vi "State_Manager.vi"(0 "Mode":enum16{"Initialize", "Manage", "Close"}(ring), 1 "Clear queue":bool, 3 "Immediate actions":bool[](array[boolean]), 4 "Reset":bool[](array[boolean]), 5 "Auto actions":bool[](array[boolean]), 6 "Config file name":path=path "C:/Users/ceslab/Documents/CES LabView/Configuration/CES_Config_test.ini", 7 "Abort action":bool) -> (8 "Spectrum type":u32, 9 "Substate":string, 10 "Action Queue":string[](array[string]), 12 "Action list":string[](array[string]), 13 "Action times":cluster{dbl[], dbl[]} {"?" format="%.2f"; "?" format="%.2f"}, 14 "Output cluster":T1, 17 "Current state":i32, 18 "Time left":dbl, 19 "error out":errorcluster)   [LabVIEW 2025]
uses:
  <vilib>/regexp/Match Regular Expression.xnode
panel:
  out "State array":i32[][](array[numeric])
  out "Action data":i32[][](array[numeric])
  out "Action count":i32[](array[numeric])
  out "Linked index":i32[](array[numeric])
  out "Mode":i32[](array[numeric])
  out "Frequency":i32[](array[numeric])
  out "Linked state":string[](array[string])
  out "Action Queue":i32[](array[numeric])
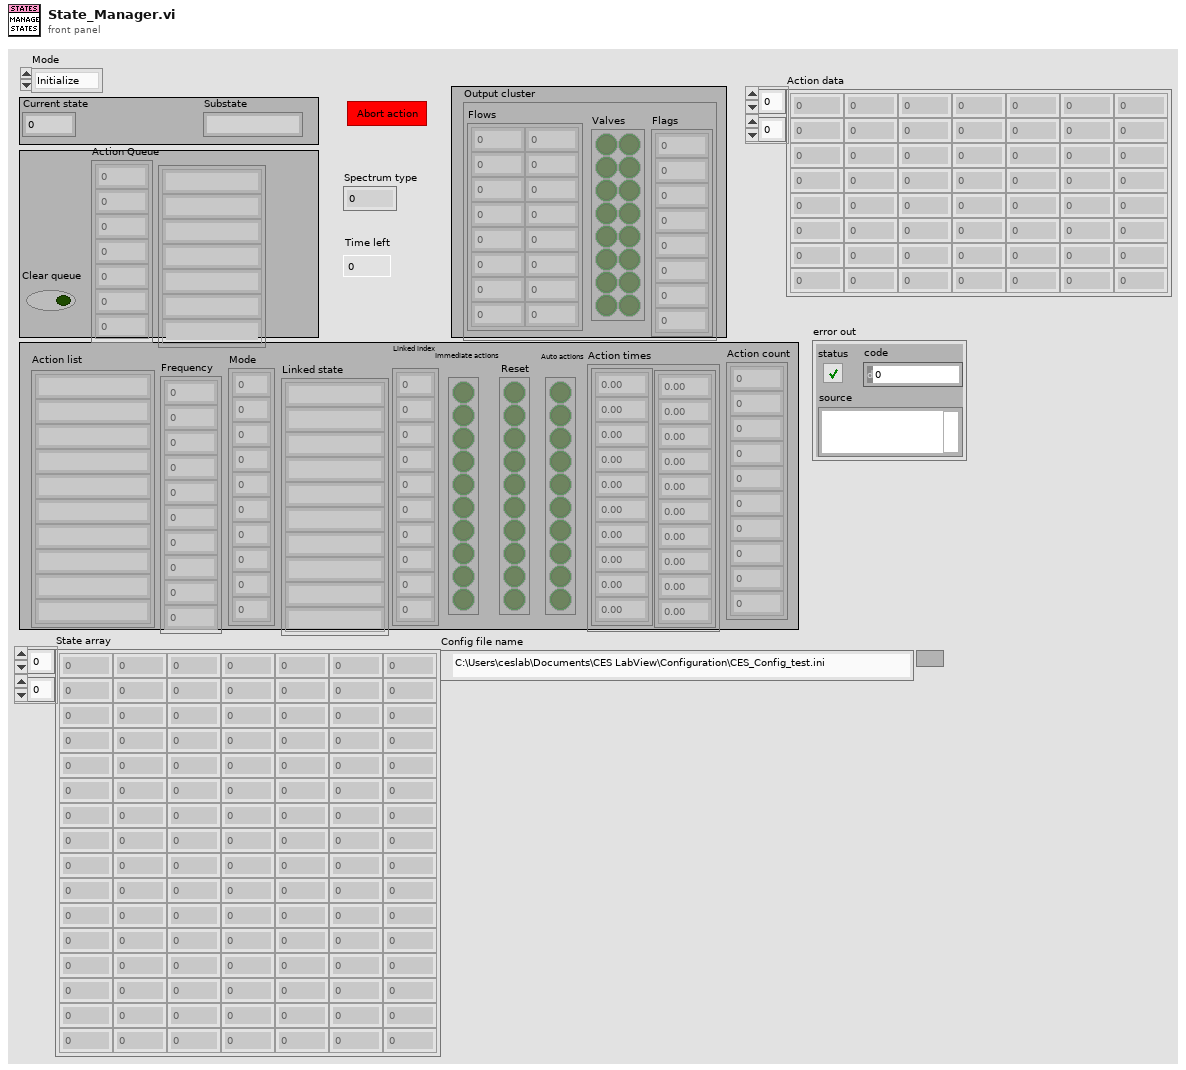
[diagram p1: front panel]
types:
  T1 = cluster{"Flows":dbl[][], "Valves":bool[][], "Flags":i32[]}
  T2 = enum16{"Spectrometer", "Calculations", "BBB", "States", "Actions"}
  T3 = cluster{"num_flags":i32, "num_flows":i32, "num_valves":i32}
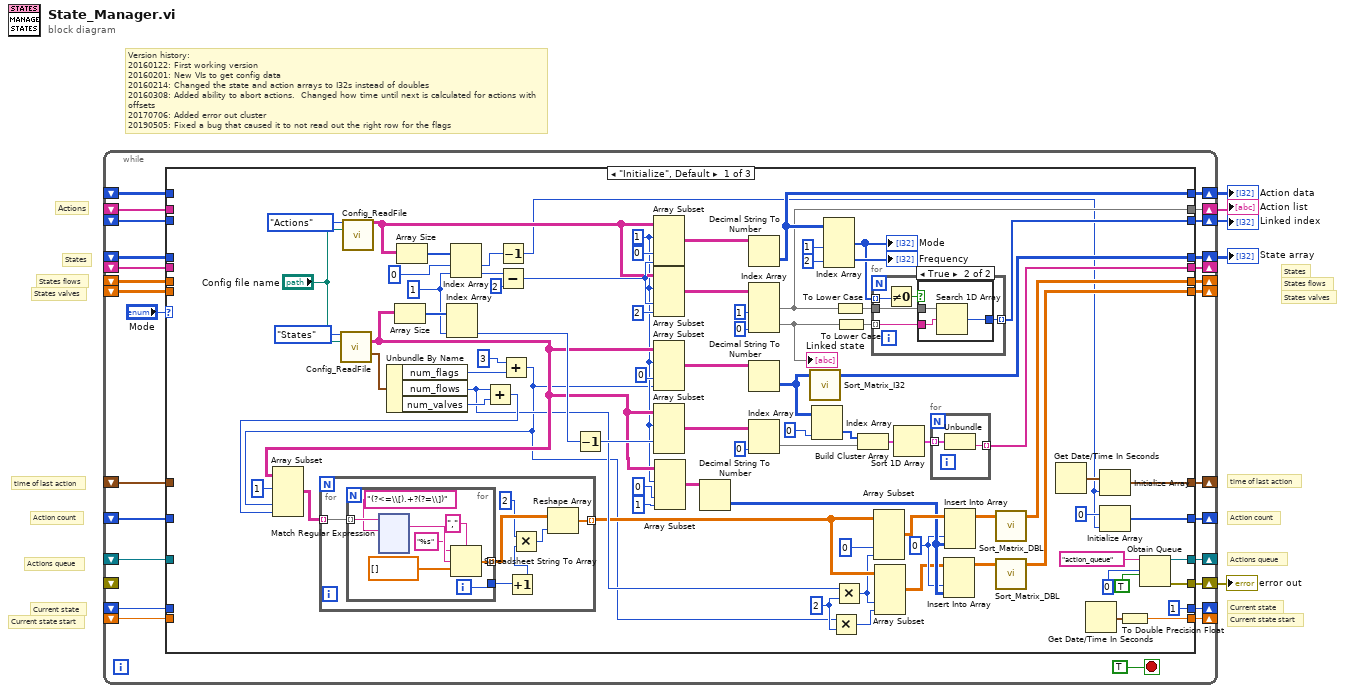
[diagram p0: block diagram]
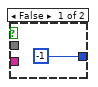
[diagram p2: hidden frame]
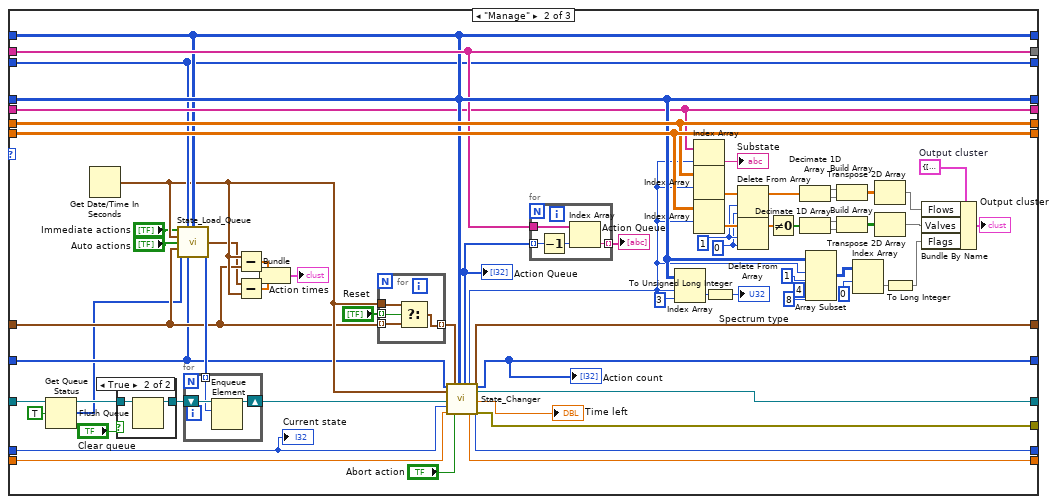
[diagram p3: hidden frame]
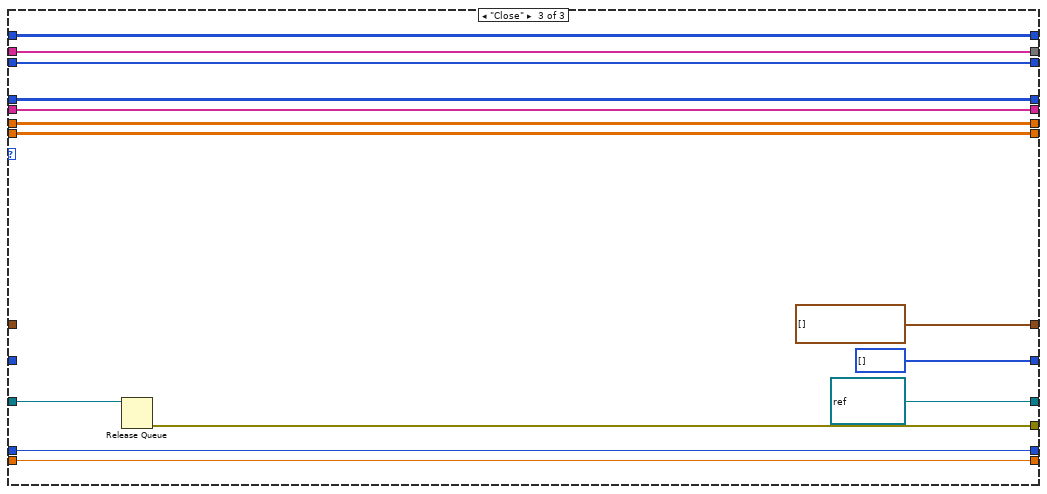
[diagram p5: hidden frame]
diagram:
  # "Version history:\n20160122: First working version\n20160201: New VIs to get config data\n20160214: Changed the state and action arrays to I32s instead of doubles\n20160308: Added ability to abort actions.  Changed how time until next is calculated for actions with offsets\n20170706: Added error out cluster\n20190505: Fixed a bug that caused it to not read out the right row for the flags"
  # "Action count"
  # "Current state start"
  # "Current state"
  # "time of last action"
  # "Actions queue"
  # "States valves"
  # "States flows"
  # "States"
  # "Actions"
  # "Action count"
  # "Current state start"
  # "Current state"
  # "time of last action"
  # "Actions queue"
  # "States valves"
  # "States flows"
  # "States"
  n1 = while {
    shift-right: [w30] -> w3
    shift-left: _ -> [w29]
    shift-right: [w28] -> w5
    shift-left: _ -> [w27]
    shift-right: [w17] -> w2
    shift-left: _ -> [w21]
    shift-right: [w26] -> _
    shift-left: _ -> [w20]
    shift-right: [w25] -> _
    shift-left: _ -> [w19]
    shift-right: [w24] -> _
    shift-left: _ -> [w18]
    shift-right: [w23] -> _
    shift-left: _ -> [w22]
    shift-right: [w16] -> _
    shift-left: _ -> [w15]
    shift-right: [w14] -> _
    shift-left: _ -> [w13]
    shift-right: [w12] -> w4
    shift-left: _ -> [w11]
    shift-right: [w9] -> _
    shift-left: _ -> [w7]
    shift-right: [w10] -> _
    shift-left: _ -> [w8]
    shift-right: [w6] -> w1
    shift-left: _ -> [_]
    stop <- TRUE stop-if-true
    n2 = case shown="\"Initialize\", Default" "Mode" {
      tunnel: [w91 w275 w352] -> w30
      tunnel: w29 -> [_ w275 w352]
      tunnel: [w81 w285 w351] -> w28
      tunnel: w27 -> [_ w285 w351]
      tunnel: [w100 w277 w349] -> w26
      tunnel: [w75 w317 w348] -> w25
      tunnel: [w74 w318 w347] -> w24
      tunnel: [w99 w282 timestamp[] []] -> w23
      tunnel: w22 -> [_ w269 _]
      tunnel: w21 -> [_ w286 w350]
      tunnel: w20 -> [_ w277 w349]
      tunnel: w19 -> [_ w317 w348]
      tunnel: w18 -> [_ w318 w347]
      tunnel: [w76 w286 w350] -> w17
      tunnel: [w95 w283 refnum<queue> refnum ("queue out")] -> w16
      tunnel: w15 -> [_ w323 w346]
      tunnel: [w92 w278 i32[] []] -> w14
      tunnel: w13 -> [_ w268 _]
      tunnel: [w85 w274 w342] -> w12
      tunnel: w11 -> [_ w274 w342]
      tunnel: [1 w260 w341] -> w10
      tunnel: [w82 w261 w340] -> w9
      tunnel: w8 -> [_ w280 w341]
      tunnel: w7 -> [_ w281 w340]
      tunnel: [w70 w259 w339] -> w6
      frame "Initialize", Default {
        w42 = 0 ("disabled index (col)")
        w39 = 2 ("y")
        w58 = 1 ("index")
        w50 = 1 ("index")
        n3 = call "Config_ReadFile.vi"("Section"=T2."States", "Config file name"="Config file name") -> ("State data"=w54:string[][], "state_elements"=w62:T3)  [unwired: 7 in, 5 out]
        n4 = call "Config_ReadFile.vi"("Section"=T2."Actions", "Config file name"="Config file name") -> ("Actions data"=w68:string[][])  [unwired: 7 in, 6 out]
        n5 = Unbundle By Name(w62) -> ("num_flags"=w61:i32, "num_flows"=w46:i32, "num_valves"=w49:i32)
        n6 = Array Size(array=w54) -> (size(s)=w69:i32[])
        n7 = Array Size(array=w68) -> (size(s)=w67:i32[])
        n8 = Index Array(array=w69, index #2=w58) -> (element #2=w57:i32)  [unwired: 1 in, 1 out]
        n9 = Index Array(array=w67, index #1=0 ("index"), index #2=w58) -> (element #1=w64:i32, element #2=w66:i32)
        n10 = Add(x=w46, y=w49) -> (x+y=w48:i32)
        n11 = Decrement(x=w64) -> (x-1=w63:i32)
        n12 = Subtract(x=w66, y=2 ("index")) -> (x-y=w72:i32)
        n13 = Add(x=3, y=w61) -> (x+y=w38:i32)
        n14 = Array Subset(array=w54, index (row)=1 ("index"), index (col)=w38, length (col)=w48) -> (w55:string[][])  [unwired: 1 in]
        n15 = for {
          tunnel: w55 -> [w121] mode=indexing
          tunnel: [w115] -> w41 mode=indexing
          n16 = for {
            tunnel: w121 -> [w129] mode=indexing
            tunnel: [w123] -> w120 mode=indexing
            tunnel: [w122] -> w116
            i -> [w122]
            n17 = xnode "Match Regular Expression"("input string"=w129, "regular expression"="(?<=\\[).+?(?=\\])") -> ("whole match"=w127:string)  [unwired: 4 in, 4 out]
            n18 = Spreadsheet String To Array(delimiter (Tab)=",", format string="%s" ("spreadsheet string"), spreadsheet string=w127, array type (2D Dbl)=dbl[] []) -> (array=w123:dbl[])
          }
          n19 = Increment(x=w116) -> (x+1=w117:i32)
          n20 = Multiply(x=2, y=w117) -> (x*y=w118:i32)
          n21 = Reshape Array(w120, w118) -> (w115:dbl[])
        }
        n22 = Decrement(x=w57) -> (x-1=w71:i32)
        n23 = Array Subset(array=w68, index (row)=w50, index (col)=0 ("index"), length (col)=w72) -> (w109:string[][])  [unwired: 1 in]
        n24 = Array Subset(array=w68, index (row)=w50, index (col)=w72, length (col)=2 ("length")) -> (w107:string[][])  [unwired: 1 in]
        n25 = Array Subset(array=w54, index (row)=w50, index (col)=0 ("index"), length (col)=w38) -> (w113:string[][])  [unwired: 1 in]
        n26 = Array Subset(array=w54, index (row)=w50, index (col)=w71) -> (w112:string[][])  [unwired: 2 in]
        n27 = Array Subset(array=w54, index (row)=w50, index (col)=0 ("index"), length (col)=1 ("length")) -> (w51:string[][])  [unwired: 1 in]
        n28 = Decimal String To Number(string=w51) -> (number=w43:i32[][])  [unwired: 2 in, 1 out]
        n29 = Decimal String To Number(string=w109) -> (number=w91:i32[][])  [unwired: 2 in, 1 out]
        n30 = Index Array(array=w107, index (col) #1=1 ("disabled index (col)"), index (col) #2=0 ("disabled index (col)")) -> (element #1=w81:string[], element #2=w79:string[])  [unwired: 2 in]
        "Linked state" <- w79
        n31 = Decimal String To Number(string=w113) -> (number=w77:i32[][])  [unwired: 2 in, 1 out]
        n32 = Index Array(array=w112, index (col)=0 ("disabled index (col)")) -> (element=w103:string[])  [unwired: 1 in]
        n33 = call "Sort_Matrix_I32.vi"("Unsort array in"=w77) -> ("Sorted array out"=w76:i32[][])  [unwired: 26 in]
        n34 = Index Array(array=w77, index (col)=0 ("disabled index (col)")) -> (element=w104:i32[])  [unwired: 1 in]
        n35 = Index Array(array=w91, index (col) #1=1 ("disabled index (col)"), index (col) #2=2 ("disabled index (col)")) -> (element #1=w86:i32[], element #2=→"Frequency":i32[])  [unwired: 2 in]
        "Mode" <- w86
        n36 = Multiply(x=w38, y=w39) -> (x*y=w37:i32)
        n37 = Multiply(x=w46, y=w39) -> (x*y=w40:i32)
        n38 = To Lower Case(string=w81) -> (all lower case string=w80:string[])
        n39 = To Lower Case(string=w79) -> (all lower case string=w78:string[])
        n40 = Build Cluster Array(w104, w103) -> (w102:cluster{"Section":i32, "Section":string}[])
        n41 = for {
          tunnel: w78 -> [w249] mode=indexing
          tunnel: w86 -> [w251] mode=indexing
          tunnel: w80 -> [w248]
          tunnel: [w247] -> w85 mode=indexing
          n42 = Not Equal To 0?(x=w251) -> (x != 0?=w250:bool)
          n43 = case shown="True" w250 {
            tunnel: w249 -> [_ w254]
            tunnel: w248 -> [_ w255]
            tunnel: [-1 w253] -> w247
            frame False {
            }
            frame True {
              n44 = Search 1D Array(1D array=w255, element=w254) -> (index of element=w253:i32)  [unwired: 1 in]
            }
          }
        }
        n45 = Array Subset(array=w41, index (col)=0 ("index"), length (col)=w40) -> (w45:dbl[][])  [unwired: 2 in]
        n46 = Array Subset(array=w41, index (col)=w40, length (col)=w37) -> (w36:dbl[][])  [unwired: 2 in]
        n47 = Sort 1D Array(array=w102) -> (sorted array=w101:cluster{"Section":i32, "Section":string}[])
        n48 = for {
          tunnel: w101 -> [w257] mode=indexing
          tunnel: [w256] -> w100 mode=indexing
          n49 = Unbundle(w257) -> ("Section"=w256:string)  [unwired: 1 out]
        }
        n50 = Insert Into Array(array=w36, index (col)=w42, new element=w43) -> (w35:dbl[][])  [unwired: 1 in]
        n51 = Insert Into Array(array=w45, index (col)=w42, new element=w43) -> (w44:dbl[][])  [unwired: 1 in]
        n52 = call "Sort_Matrix_DBL.vi"("Unsort array in"=w44) -> ("Sorted array out"=w75:dbl[][])  [unwired: 26 in]
        n53 = call "Sort_Matrix_DBL.vi"("Unsort array in"=w35) -> ("Sorted array out"=w74:dbl[][])  [unwired: 26 in]
        n54 = Get Date/Time In Seconds() -> (seconds since 1Jan1904=w94:timestamp)
        n55 = Get Date/Time In Seconds() -> (seconds since 1Jan1904=w84:timestamp)
        n56 = Initialize Array(w94, w63) -> (w99:timestamp[])
        n57 = Initialize Array(0, w63) -> (w92:i32[])
        n58 = To Double Precision Float(number=w84) -> (double precision float=w82:dbl)
        n59 = Obtain Queue(name (unnamed)="action_queue", element data type=0, create if not found? (T)=TRUE) -> (queue out=w95:refnum<queue>, error out=w70:errorcluster)  [unwired: 2 in, 1 out]
      }
      frame "Manage" {
        w302 = T1 {"Flows"=[], "Valves"=[], "Flags"=[]}  # Output cluster
        w313 = 1
        w312 = 0
        n60 = Get Queue Status(queue=w323, return elements? (F)=TRUE) -> (queue out=w322:refnum<queue>, elements=w267:i32[])  [unwired: 1 in, 6 out]
        n61 = Get Date/Time In Seconds() -> (seconds since 1Jan1904=w271:timestamp)
        n62 = case shown="True" "Clear queue" {
          tunnel: w322 -> [w336 w338]
          tunnel: [w336 w337] -> w320
          frame False {
          }
          frame True {
            n63 = Flush Queue(queue=w338) -> (queue out=w337:refnum<queue>)  [unwired: 1 in, 2 out]
          }
        }
        n64 = call "State_Load_Queue.vi"("Immediate actions in"="Immediate actions", "Linked index"=w274, "Actions"=w275, "Current time"=w271, "Auto actions in"="Auto actions", "Time of last action"=w269, "Queue in"=w267, "Action count in"=w268) -> ("Time til next out"=w266:timestamp[], "Actions for queue"=w273:i32[])  [unwired: 6 in]
        n65 = for {
          shift-right: [w334] -> w284
          shift-left: w320 -> [w335]
          tunnel: w273 -> [w333] mode=indexing
          n66 = Enqueue Element(queue=w335, element=w333) -> (queue out=w334:refnum<queue>)  [unwired: 2 in, 2 out]
        }
        n67 = Subtract(x=w271, y=w269) -> (x-y=w291:dbl[])
        n68 = Subtract(x=w266, y=w271) -> (x-y=w290:dbl[])
        n69 = Bundle(w291, w290) -> (→"Action times":cluster{dbl[], dbl[]})  [unwired: 1 in]
        n70 = for {
          tunnel: w269 -> [w330] mode=indexing
          tunnel: "Reset" -> [w332] mode=indexing
          tunnel: w271 -> [w331]
          tunnel: [w329] -> w287 mode=indexing
          n71 = Select(t=w331, s=w332, f=w330) -> (s? t:f=w329:timestamp)
        }
        n72 = call "State_Changer.vi"("Action count in"=w268, "Time in"=w271, "Action queue in"=w284, "Current state in"=w280, "Current state start in"=w281, "Time of last action in"=w287, "Abort action"="Abort action", "States"=w286, "Actions"=w275) -> ("Action Queue"=w279:i32[], "Current state index"=w258:i32, "Current state start out"=w261:dbl, "Action count out"=w278:i32[], "Action Queue out"=w283:refnum<queue>, "Time of last action out"=w282:timestamp[], "Time left"=→"Time left":dbl, "Current state out"=w260:i32, "error out"=w259:errorcluster)  [unwired: 2 in]
        "Action Queue" <- w279
        "Action count" <- w278
        n73 = for {
          tunnel: w279 -> [w326] mode=indexing
          tunnel: w285 -> [w328]
          tunnel: [w325] -> w288 mode=indexing
          n74 = Decrement(x=w326) -> (x-1=w327:i32)
          n75 = Index Array(array=w328, index=w327) -> (element=w325:string)
        }
        "Action Queue" <- w288
        n76 = Index Array(array=w286, index (row)=w258, index (col)=3 ("disabled index (col)")) -> (element=w265:i32)
        n77 = Index Array(array=w277, index=w258) -> (element=→"Substate":string)
        n78 = Index Array(array=w317, index (row)=w258) -> (element=w315:dbl[])  [unwired: 1 in]
        n79 = Index Array(array=w318, index (row)=w258) -> (element=w314:dbl[])  [unwired: 1 in]
        n80 = To Unsigned Long Integer(number=w265) -> (unsigned 32bit integer=→"Spectrum type":u32)
        n81 = Delete From Array(array=w315, length=w313, index=w312) -> (array with subset deleted=w303:dbl[])  [unwired: 1 out]
        n82 = Delete From Array(array=w314, length=w313, index=w312) -> (array with subset deleted=w311:dbl[])  [unwired: 1 out]
        n83 = Not Equal To 0?(x=w311) -> (x != 0?=w304:bool[])
        n84 = Decimate 1D Array(w303) -> (w310:dbl[], w309:dbl[])
        n85 = Decimate 1D Array(w304) -> (w307:bool[], w306:bool[])
        n86 = Array Subset(array=w286, index (row)=w258, length (row)=1, index (col)=4 ("index"), length (col)=8 ("length")) -> (w295:i32[][])
        n87 = Build Array(w310, w309) -> (w308:dbl[][])
        n88 = Build Array(w307, w306) -> (w305:bool[][])
        n89 = Index Array(array=w295, index (row)=0) -> (element=w292:i32[])  [unwired: 1 in]
        n90 = Transpose 2D Array(2D array=w308) -> (transposed array=w301:dbl[][])
        n91 = Transpose 2D Array(2D array=w305) -> (transposed array=w300:bool[][])
        n92 = To Long Integer(number=w292) -> (32bit integer=w293:i32[])
        n93 = Bundle By Name(cluster=w302, "Flows"=w301, "Valves"=w300, "Flags"=w293) -> (→"Output cluster":T1)
        "Current state" <- w280
      }
      frame "Close" {
        n94 = Release Queue(queue=w346) -> (error out=w339:errorcluster)  [unwired: 2 in, 2 out]
      }
    }
  }
  "Action list" <- w5
  "Linked index" <- w4
  "Action data" <- w3
  "State array" <- w2
  "error out" <- w1
